vi "ConvertMFCBytes.vi"(1 "Device Input Cluster":T1={"Dnet"="", "Node"=0, "Type"="", "ID Number"=0, "SCCM"=0.0, "FullScale"=0.0, "Input Bytes"=0, "Output Bytes"=0, "Input Start Location"=0, "Output Start Location"=0, "Enabled"=TRUE, "Bytes"=[]}) -> (0 "Device Output Cluster":T1={"Dnet"="", "Node"=0, "Type"="", "ID Number"=0, "SCCM"=0.0, "FullScale"=0.0, "Input Bytes"=0, "Output Bytes"=0, "Input Start Location"=0, "Output Start Location"=0, "Enabled"=TRUE, "Bytes"=[]})   [LabVIEW 2011]
uses:
  GlobalVariables.vi
  Controls/Device Cluster.ctl
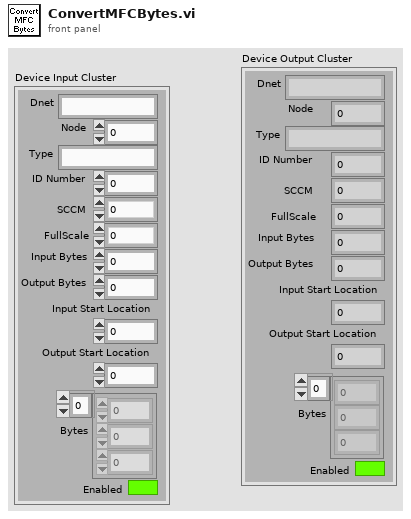
[diagram p1: front panel]
types:
  T1 = typedef "Device Cluster.ctl" = cluster{"Dnet":string, "Node":i32, "Type":string, "ID Number":u8, "SCCM":dbl, "FullScale":dbl, "Input Bytes":i32, "Output Bytes":i32, "Input Start Location":i32, "Output Start Location":i32, "Enabled":bool, "Bytes":u8[]}
  T2 = cluster{"[0]":u8, "[1]":u8, "[2]":u8, "[3]":u8, "[4]":u8, "[5]":u8, "[6]":u8, "[7]":u8}
  T3 = typedef "MFC Cluster.ctl" = cluster{"ID Number":u8, "Status":bool[], "Flow (SCCM)":dbl, "SetPoint (SCCM)":dbl, "Actuator Override":i8, "Actuator Drive Valve":i16, "Setpoint Output":dbl}
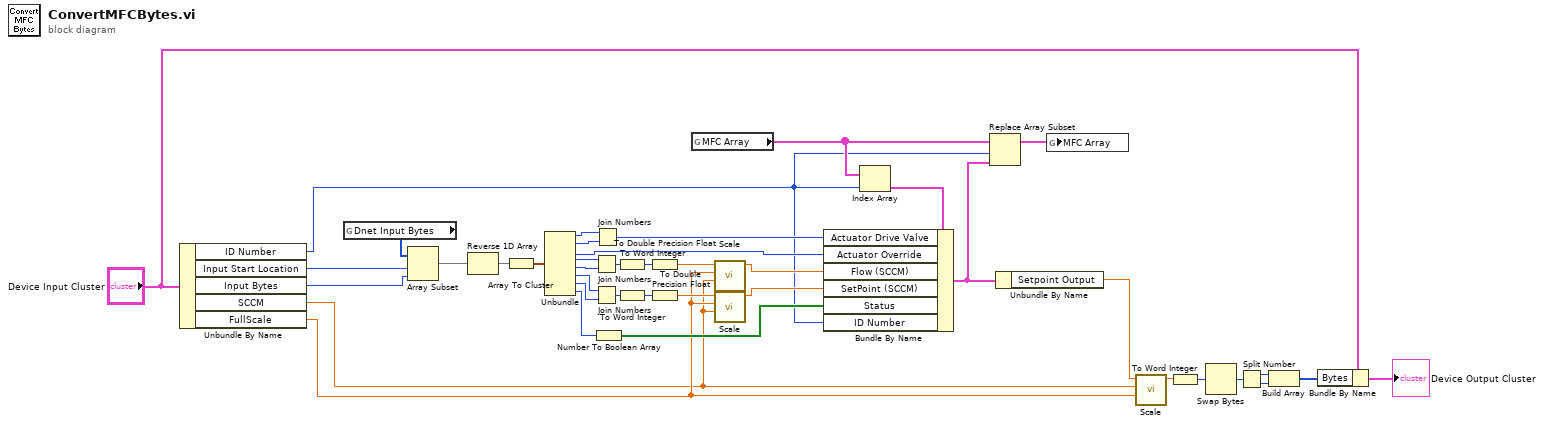
[diagram p0: block diagram]
diagram:
  n1 = Unbundle By Name("Device Input Cluster") -> ("ID Number"=w2:u8, "Input Start Location"=w3:i32, "Input Bytes"=w4:i32, "SCCM"=w5:dbl, "FullScale"=w6:dbl)
  n2 = global read "GlobalVariables.vi" "Dnet Input Bytes"() -> (w27:u8[])
  n3 = Array Subset(array=w27, index=w3, length=w4) -> (w26:u8[])
  n4 = Reverse 1D Array(array=w26) -> (reversed array=w39:u8[])
  n5 = Array To Cluster(array=w39) -> (cluster=w40:T2)
  n6 = Unbundle(w40) -> ("[0]"=w32:u8, "[1]"=w33:u8, "[2]"=w24:u8, "[3]"=w34:u8, "[4]"=w35:u8, "[5]"=w36:u8, "[6]"=w37:u8, "[7]"=w38:u8)
  n7 = Join Numbers(hi=w34, lo=w35) -> ((hi.lo)=w28:u16)
  n8 = Join Numbers(hi=w36, lo=w37) -> ((hi.lo)=w29:u16)
  n9 = Join Numbers(hi=w32, lo=w33) -> ((hi.lo)=w23:u16)
  n10 = Number To Boolean Array(number=w38) -> (Boolean array=w25:bool[])
  n11 = To Word Integer(number=w28) -> (16bit integer=w31:i16)
  n12 = To Word Integer(number=w29) -> (16bit integer=w30:i16)
  n13 = To Double Precision Float(number=w31) -> (double precision float=w17:dbl)
  n14 = To Double Precision Float(number=w30) -> (double precision float=w16:dbl)
  n15 = global read "GlobalVariables.vi" "MFC Array"() -> (w19:T3[])
  n16 = call "Scale.vi"("Factor"=w5, "FullScale"=w6, "Input"=w17) -> ("Output"=w15:dbl)  [unwired: 8 in]
  n17 = call "Scale.vi"("Factor"=w5, "FullScale"=w6, "Input"=w16) -> ("Output"=w14:dbl)  [unwired: 8 in]
  n18 = Index Array(array=w19, index=w2) -> (element=w21:T3)
  n19 = Bundle By Name(cluster=w21, "Actuator Drive Valve"=w23, "Actuator Override"=w24, "Flow (SCCM)"=w15, "SetPoint (SCCM)"=w14, "Status"=w25, "ID Number"=w2) -> (w20:T3)
  n20 = Replace Array Subset(array=w19, new element=w20, index=w2) -> (w18:T3[])
  n21 = Unbundle By Name(w20) -> ("Setpoint Output"=w7:dbl)
  n22 = global write "GlobalVariables.vi" "MFC Array"(w18) -> ()
  n23 = call "Scale.vi"("Factor"=w6, "FullScale"=w5, "Input"=w7) -> ("Output"=w13:dbl)  [unwired: 8 in]
  n24 = To Word Integer(number=w13) -> (16bit integer=w12:i16)
  n25 = Swap Bytes(anything=w12) -> (byte swapped=w11:i16)
  n26 = Split Number(x=w11) -> (hi(x)=w9:u8, lo(x)=w10:u8)
  n27 = Build Array(w9, w10) -> (w8:u8[])
  n28 = Bundle By Name(cluster="Device Input Cluster", "Bytes"=w8) -> (→"Device Output Cluster":T1)
